vi "OFBS_test_ANN.vi"(6 "Test Data":T1, 8 "error in (no error)":errorcluster, 9 "ANN in":T2={"Training Data"={"dim in"=0, "dim out"=0, "# samples"=0, "Input"=[], "Output"=[]}, "Normalize Info"={"input min"=[], "input max"=[], "output min"=[], "output max"=[]}, "3-layer NN"={"# input neuron "=0, "# hidden neuron"=0, "# output neuron"=0, "Weight (I->H)"=[], "Weight (H->O)"=[], "Output"=[], "Hidden Out"=[], "Derivation Output"=[], "Derivation Hidden"=[], "dw (I->H)"=[], "dw (H->O)"=[]}, "Ternimal Condition"={"min MSE"=1e-05, "min delta MSE"=1e-05, "min step length"=1e-08, "max iteration"=inf}}, 10 "Parameters":i32[](array[numeric]), 11 "OFBS class in":refnum<class "OptFreqBandsSearch.lvclass">) -> (0 "error out":errorcluster, 1 "Confusion Matrix":i32[][](array[numeric]), 2 "Accuracy":dbl, 3 "OFBS class out":refnum<class "OptFreqBandsSearch.lvclass">)   [LabVIEW 2016, in "Optimal Frequency Bands Search.lvlib" / "OptFreqBandsSearch.lvclass"]
doc: "Метод, реализующий тестирование классификатора на основе многослойного персептрона. Для тестирования могут использоваться обучающие, либо тестовые данные"
uses:
  OptFreqBandsSearch.lvclass
  <vilib>/addons/Machine Learning/Supervised Learning/ml_BP_Project.ctl
  <vilib>/addons/Machine Learning/Supervised Learning/ml_BP_Data.ctl
  <vilib>/addons/Machine Learning/Supervised Learning/ml_BP_Normalize Data.ctl
  <vilib>/addons/Machine Learning/Supervised Learning/ml_BP_3layer Feedforward.ctl
  <vilib>/addons/Machine Learning/Supervised Learning/ml_BP_Terminal Condition.ctl
  OFBS_DataTypes.ctl
  OptFreqBandsSearch.lvclass/OptFreqBandsSearch.ctl
  4. Accuracy Assessment for EEG Classification/_vlib/CU_CohenKappa.vi
  Optimal Frequency Bands Search.lvlib
  <vilib>/addons/Machine Learning/NILabs_MLT.lvlib
  4. Accuracy Assessment for EEG Classification/Classifier.lvlib
panel:
  # "This VI is a part of BCI Design library, http://www.ru-bci.org \nCopyright © 2020, Sotnikov Peter, All rights reserved. License: CC BY-NC 4.0"
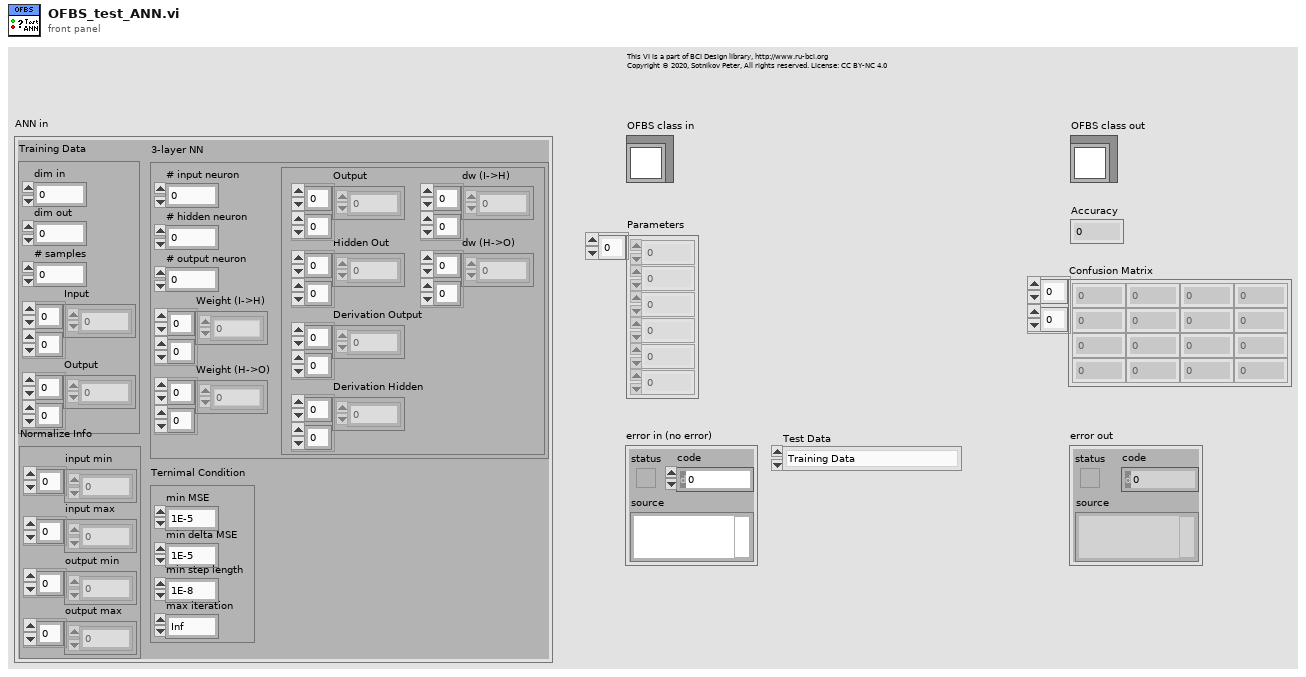
[diagram p1: front panel]
types:
  T1 = typedef "Optimal Frequency Bands Search.lvlib/OFBS_DataTypes.ctl" = enum16{"Training Data", "Test Data", "Training Data (cross-check)", "Test Data (cross-check)"}
  T2 = typedef "NILabs_MLT.lvlib/ml_BP_Project.ctl" = cluster{"Training Data":T3, "Normalize Info":T4, "3-layer NN":T5, "Ternimal Condition":T6}
  T3 = typedef "NILabs_MLT.lvlib/ml_BP_Data.ctl" = cluster{"dim in":i32, "dim out":i32, "# samples":i32, "Input":dbl[][], "Output":dbl[][]}
  T4 = typedef "NILabs_MLT.lvlib/ml_BP_Normalize Data.ctl" = cluster{"input min":dbl[], "input max":dbl[], "output min":dbl[], "output max":dbl[]}
  T5 = typedef "NILabs_MLT.lvlib/ml_BP_3layer Feedforward.ctl" = cluster{"# input neuron ":i32, "# hidden neuron":i32, "# output neuron":i32, "Weight (I->H)":dbl[][], "Weight (H->O)":dbl[][], "Output":dbl[][], "Hidden Out":dbl[][], "Derivation Output":dbl[][], "Derivation Hidden":dbl[][], "dw (I->H)":dbl[][], "dw (H->O)":dbl[][]}
  T6 = typedef "NILabs_MLT.lvlib/ml_BP_Terminal Condition.ctl" = cluster{"min MSE":dbl, "min delta MSE":dbl, "min step length":dbl, "max iteration":dbl}
  T7 = typedef "Classifier.lvlib/CU_ClassifierQualityMeasure.ctl" = enum16{"Accuracy", "Cohen's kappa"}
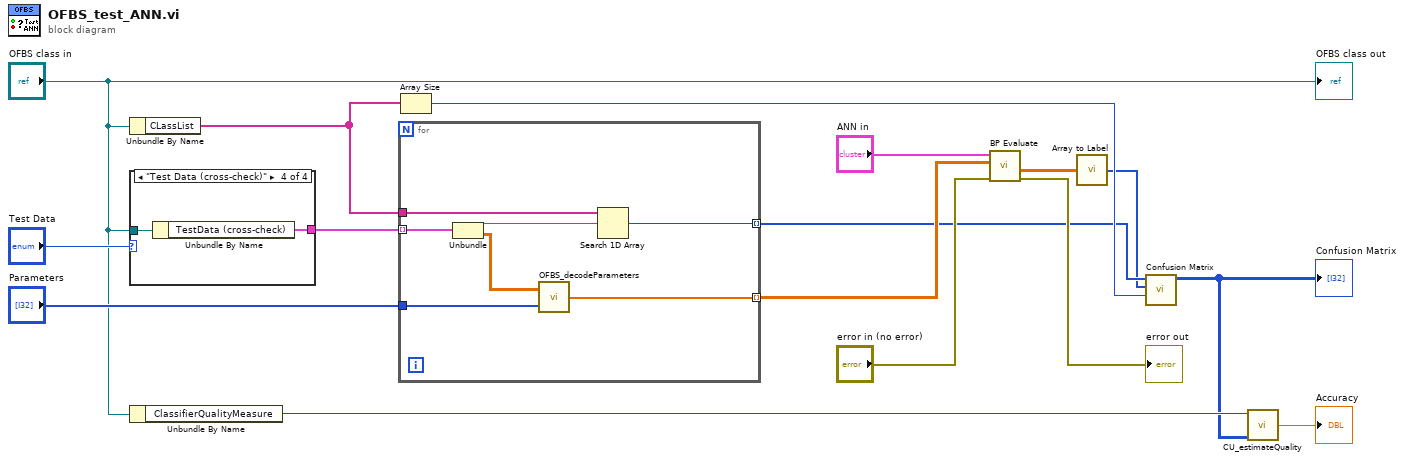
[diagram p0: block diagram]
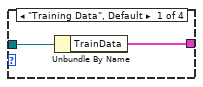
[diagram p2: hidden frame]
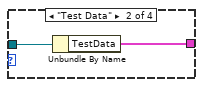
[diagram p3: hidden frame]
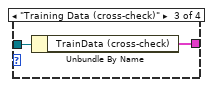
[diagram p4: hidden frame]
diagram:
  n1 = Unbundle By Name("OFBS class in") -> ("CLassList"=w6:string[])
  n2 = case shown="\"Test Data (cross-check)\"" "Test Data" {
    tunnel: "OFBS class in" -> [w18 w20 w22 w24]
    tunnel: [w17 w19 w21 w23] -> w5
    frame "Training Data", Default {
      n3 = Unbundle By Name(w18) -> ("TrainData"=w17:cluster{"ClassLabel":string, "Trial":dbl[][]}[])
    }
    frame "Test Data" {
      n4 = Unbundle By Name(w20) -> ("TestData"=w19:cluster{"ClassLabel":string, "Trial":dbl[][]}[])
    }
    frame "Training Data (cross-check)" {
      n5 = Unbundle By Name(w22) -> ("TrainData (cross-check)"=w21:cluster{"ClassLabel":string, "Trial":dbl[][]}[])
    }
    frame "Test Data (cross-check)" {
      n6 = Unbundle By Name(w24) -> ("TestData (cross-check)"=w23:cluster{"ClassLabel":string, "Trial":dbl[][]}[])
    }
  }
  n7 = Unbundle By Name("OFBS class in") -> ("ClassifierQualityMeasure"=w4:T7)
  n8 = for {
    tunnel: w5 -> [w31] mode=indexing
    tunnel: "Parameters" -> [w29]
    tunnel: w6 -> [w28]
    tunnel: [w26] -> w9 mode=indexing
    tunnel: [w25] -> w14 mode=indexing
    n9 = Unbundle(w31) -> ("ClassLabel"=w27:string, "Trial"=w30:dbl[][])
    n10 = call "OFBS_decodeParameters.vi"("Parameters"=w29, "Trial"=w30) -> ("FeatureVector"=w25:dbl[])
    n11 = Search 1D Array(1D array=w28, element=w27) -> (index of element=w26:i32)  [unwired: 1 in]
  }
  n12 = Array Size(array=w6) -> (size(s)=w10:i32)
  n13 = call <vilib>:"BP Evaluate.vi"("error in (no error)"="error in (no error)", "Test data samples"=w14, "BP Project"="ANN in") -> ("error out"=→"error out":errorcluster, "NN outputs"=w12:dbl[][])  [unwired: 4 in, 3 out]
  n14 = call <vilib>:"Array to Label.vi"("Array"=w12) -> ("Classes"=w8:i32[])
  n15 = call <vilib>:"Confusion Matrix.vi"("# of classes"=w10, "Predicted class labels"=w8, "Actual class labels"=w9) -> ("Confusion Matrix"=w1:i32[][])  [unwired: 7 in, 1 out]
  "Confusion Matrix" <- w1
  n16 = call "CU_estimateQuality.vi"("Quality Measure in"=w4, "Confusion Matrix in"=w1) -> ("Classification Quality out"=→"Accuracy":dbl)  [unwired: 6 in]
  "OFBS class out" <- "OFBS class in"
